vi "Initialize Sensors TA.vi"(11 "?":T1={"     Use ?\nOff       On"=[FALSE, TRUE, FALSE, TRUE], "Mode:"=FALSE, "Hokuyo Port"="COM7", "Tx Prop  Port"="COM6", "Compass Port"="", "GPS Port"="", "Rx Prop  Port"="COM6"}) -> (3 "?":T1={"     Use ?\nOff       On"=[FALSE, TRUE, FALSE, TRUE], "Mode:"=FALSE, "Hokuyo Port"="COM7", "Tx Prop  Port"="COM6", "Compass Port"="", "GPS Port"="", "Rx Prop  Port"="COM6"})   [LabVIEW 2014]
uses:
  Initialize-Standard.vi
  Hokuyo URG Series.lvlib
panel:
  in  "Checksum":bool
  in  "ID Query?":bool=TRUE
  in  "Protocol":u32(ring)=2 items=["Convert to Latest", "SCIP 1.1", "SCIP 2.0"]
  # "Initialize Sensors TA"
  # "Input:"
  # "Output:"
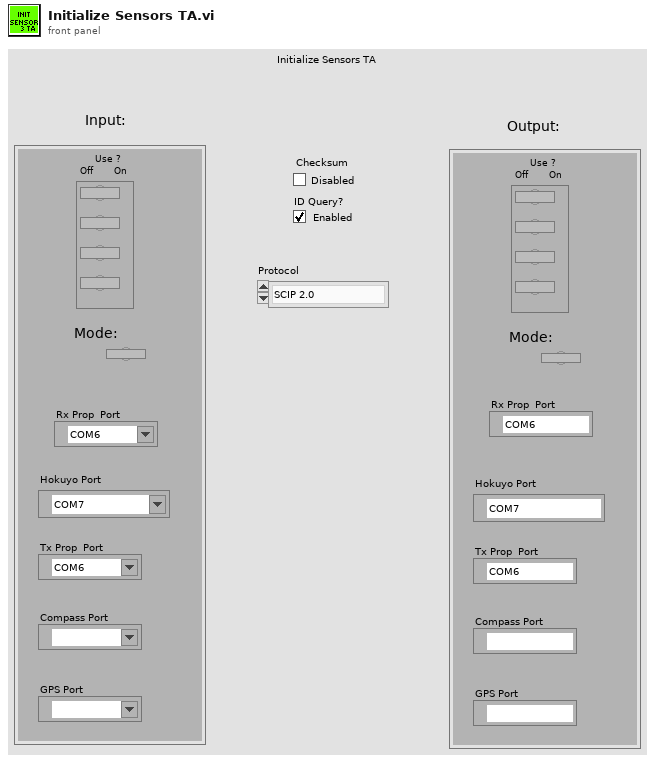
[diagram p1: front panel]
types:
  T1 = cluster{"     Use ?\nOff       On":bool[], "Mode:":bool, "Hokuyo Port":refnum<visa-resource-name>, "Tx Prop  Port":refnum<visa-resource-name>, "Compass Port":refnum<visa-resource-name>, "GPS Port":refnum<visa-resource-name>, "Rx Prop  Port":refnum<visa-resource-name>}
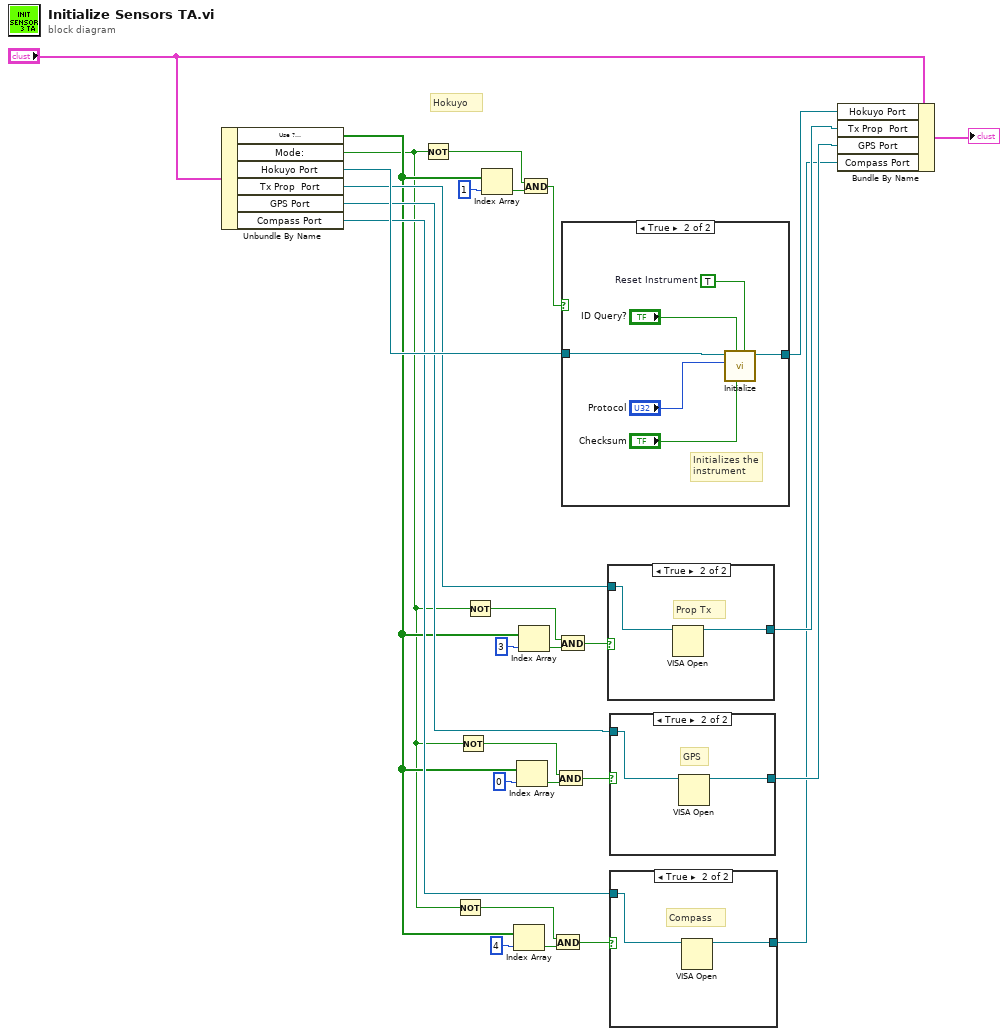
[diagram p0: block diagram]
diagram:
  # "Hokuyo"
  n1 = Unbundle By Name("?") -> ("Use ?\nOff       On"=w3:bool[], "Mode:"=w1:bool, "Hokuyo Port"=w25:refnum<visa-resource-name>, "Tx Prop  Port"=w17:refnum<visa-resource-name>, "GPS Port"=w11:refnum<visa-resource-name>, "Compass Port"=w5:refnum<visa-resource-name>)
  n2 = Not(x=w1) -> (.not. x?=w26:bool)
  n3 = Not(x=w1) -> (.not. x?=w7:bool)
  n4 = Not(x=w1) -> (.not. x?=w13:bool)
  n5 = Not(x=w1) -> (.not. x?=w2:bool)
  n6 = Index Array(array=w3, index=1) -> (element=w27:bool)
  n7 = Index Array(array=w3, index=4) -> (element=w8:bool)
  n8 = Index Array(array=w3, index=0) -> (element=w14:bool)
  n9 = Index Array(array=w3, index=3) -> (element=w19:bool)
  n10 = And(x=w26, y=w27) -> (x .and. y?=w24:bool)
  n11 = And(x=w7, y=w8) -> (x .and. y?=w6:bool)
  n12 = And(x=w13, y=w14) -> (x .and. y?=w12:bool)
  n13 = And(x=w2, y=w19) -> (x .and. y?=w18:bool)
  n14 = case shown="True" w24 {
    tunnel: w25 -> [w29 w31]
    tunnel: [w29 w30] -> w23
    frame False {
    }
    frame True {
      w33 = TRUE  # Reset Instrument
      # "Initializes the instrument"
      n15 = call-poly "Initialize.vi"("Reset? (F: No)"=w33, "Checksum (Disabled)"="Checksum", "ID Query? (Enabled)"="ID Query?", "Protocol (2: SCIP 2.0)"="Protocol", "VISA resource name"=w31) -> ("VISA resource name out"=w30:refnum<visa-resource-name>)  [unwired: 5 in, 1 out]
    }
  }
  n16 = case shown="True" w18 {
    tunnel: w17 -> [w36 w38]
    tunnel: [w36 w37] -> w16
    frame False {
    }
    frame True {
      # "Prop Tx"
      n17 = VISA Open(VISA resource name=w38) -> (VISA resource name=w37:refnum<visa-resource-name>)  [unwired: 4 in, 1 out]
    }
  }
  n18 = case shown="True" w12 {
    tunnel: w11 -> [w39 w41]
    tunnel: [w39 w40] -> w10
    frame False {
    }
    frame True {
      # "GPS"
      n19 = VISA Open(VISA resource name=w41) -> (VISA resource name=w40:refnum<visa-resource-name>)  [unwired: 4 in, 1 out]
    }
  }
  n20 = case shown="True" w6 {
    tunnel: w5 -> [w42 w44]
    tunnel: [w42 w43] -> w4
    frame False {
    }
    frame True {
      # "Compass"
      n21 = VISA Open(VISA resource name=w44) -> (VISA resource name=w43:refnum<visa-resource-name>)  [unwired: 4 in, 1 out]
    }
  }
  n22 = Bundle By Name(cluster="?", "Hokuyo Port"=w23, "Tx Prop  Port"=w16, "GPS Port"=w10, "Compass Port"=w4) -> (→"?":T1)
